vi "To String.vi"(8 "error in (no error)":errorcluster, 11 "Time Stamp in":refnum<class "Time Stamp.lvclass">) -> (0 "error out":errorcluster, 2 "String":string)   [LabVIEW 2020, in "Data.lvlib" / "Time Stamp.lvclass"]
doc: "Convert 'Generic Data in' to a string. \nThis implementation converts the TIme Stamp into a string formatted as: YYYY-MM-DD hh:mm:ss.ddd"
uses:
  Time Stamp.lvclass
  Time Stamp.lvclass/Time Stamp.ctl
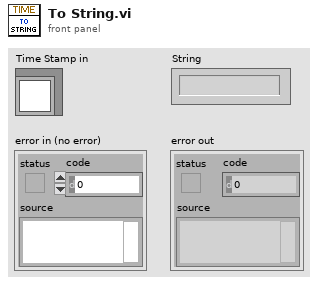
[diagram p1: front panel]
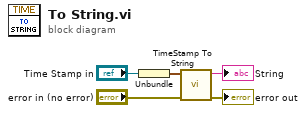
[diagram p0: block diagram]
diagram:
  n1 = Unbundle("Time Stamp in") -> (w4:timestamp)
  n2 = call "TimeStamp To String.vi"("error in (no error)"="error in (no error)", "Time Stamp"=w4) -> ("error out"=→"error out":errorcluster, "Time string"=→"String":string)  [unwired: 8 in]
